vi "Get Serial Settings.vi"(8 "error in (no error)":errorcluster, 11 "Item Ref in":T4 format="%.0x") -> (0 "error out":errorcluster, 1 "baud rate":u32=9600, 2 "VISA resource name":refnum<visa-resource-name>, 3 "Item Ref out":T4 format="%.0x", 4 "parity (even)":T1=2 items=["None", "Odd", "Even", "Mark", "Space"], 5 "serial type":T2, 6 "Wire Mode":i32(ring)=-1 items=["Unknown"=-1, "RS485/Wire4"=0, "RS485/Wire2-EchoDTR"=1, "RS485/Wire2-CtrlDTR"=2, "RS485/Wire2-Auto"=3, "RS232/DTE"=128, "RS232/DCE"=129, "RS232/AUTO"=130], 7 "flow control (none)":T3 items=["None", "XON/XOFF", "RTS/CTS", "XON/XOFF & RTS/CTS", "DTR/DSR", "XON/XOFF & DTR/DSR"])   [LabVIEW 2020, in "Modbus Master System Explorer.lvlib"]
uses:
  Modbus Master System Explorer.lvlib
  <vilib>/NI VeriStand/Custom Device API/Custom Device Item Ref.ctl
  Shared/Controls/Flow Control.ctl
  Shared/Controls/Serial Type.ctl
  Shared/Controls/Parity.ctl
  Shared/Constants.vi
  <vilib>/NI VeriStand/Custom Device API/Get Item Property (String).vi
  <vilib>/NI VeriStand/Custom Device API/Get Item Property (U32).vi
  <vilib>/NI VeriStand/Custom Device API/Get Item Property (U16).vi
  <vilib>/NI VeriStand/Custom Device API/Get Item Property (I32).vi
  Shared/Modbus Master Shared.lvlib
  <vilib>/NI VeriStand/Custom Device API/Custom Device API.lvlib
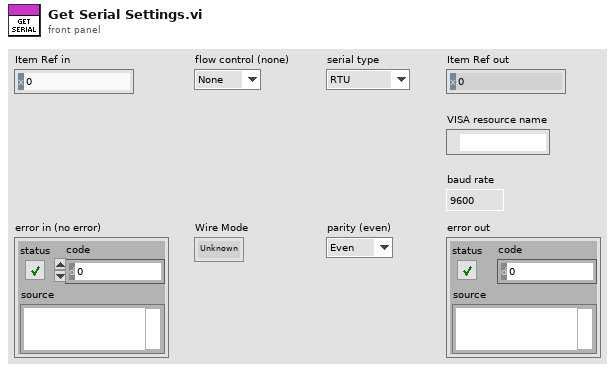
[diagram p1: front panel]
types:
  T1 = typedef "Modbus Master Shared.lvlib/Parity.ctl" = u16
  T2 = typedef "Modbus Master Shared.lvlib/Serial Type.ctl" = enum16{"RTU", "ASCII"}
  T3 = typedef "Modbus Master Shared.lvlib/Flow Control.ctl" = u16
  T4 = typedef "Custom Device API.lvlib/Custom Device Item Ref.ctl" = u64
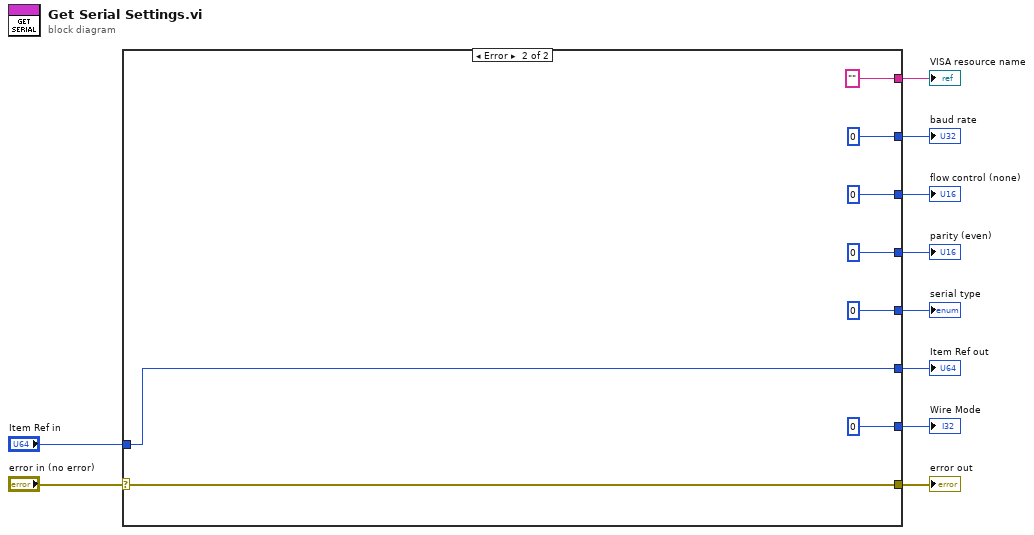
[diagram p0: block diagram]
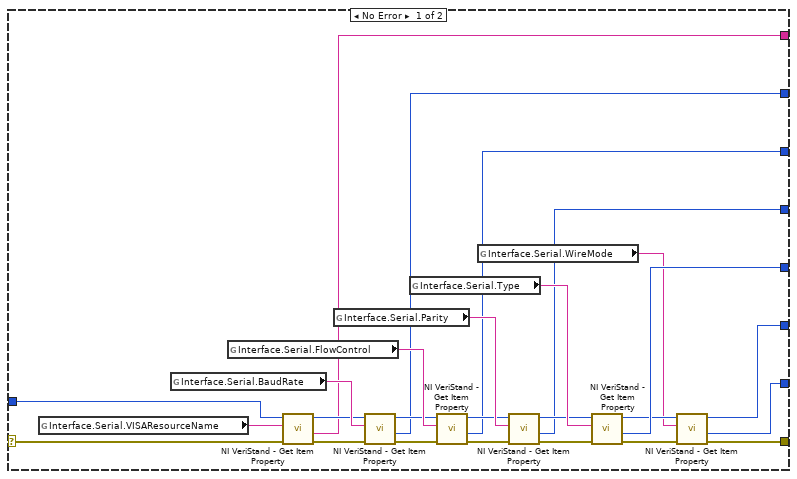
[diagram p2: hidden frame]
diagram:
  n1 = case shown="Error" "error in (no error)" {
    selector: "error in (no error)" -> [w24 w43]
    tunnel: [w11 w43] -> w10
    tunnel: [w14 w44] -> w9
    tunnel: "Item Ref in" -> [w23 w44]
    tunnel: [w21 "" ("Value")] -> w6
    tunnel: [w20 u32 0 ("Value")] -> w5
    tunnel: [w19 u16 0 ("Value")] -> w4
    tunnel: [w18 u16 0 ("Value")] -> w3
    tunnel: [w17 u16 0 ("Value")] -> w2
    tunnel: [w13 0 ("Value")] -> w1
    frame No Error {
      n2 = global read "Constants.vi" "Interface.Serial.VISAResourceName"() -> (w22:string)
      n3 = global read "Constants.vi" "Interface.Serial.BaudRate"() -> (w27:string)
      n4 = global read "Constants.vi" "Interface.Serial.FlowControl"() -> (w30:string)
      n5 = call-poly <vilib>:"NI VeriStand - Get Item Property.vi"("error in (no error)"=w24, "Property Name"=w22, "Item Ref in"=w23) -> ("error out"=w25:errorcluster, "Value"=w21:string, "Item Ref out"=w26:T4)  [unwired: 5 in, 1 out]
      n6 = global read "Constants.vi" "Interface.Serial.Parity"() -> (w33:string)
      n7 = call-poly <vilib>:"NI VeriStand - Get Item Property.vi"("error in (no error)"=w25, "Property Name"=w27, "Item Ref in"=w26) -> ("error out"=w28:errorcluster, "Value"=w20:u32, "Item Ref out"=w29:T4)  [unwired: 5 in, 1 out]
      n8 = global read "Constants.vi" "Interface.Serial.Type"() -> (w36:string)
      n9 = call-poly <vilib>:"NI VeriStand - Get Item Property.vi"("error in (no error)"=w28, "Property Name"=w30, "Item Ref in"=w29) -> ("error out"=w31:errorcluster, "Value"=w19:u16, "Item Ref out"=w32:T4)  [unwired: 5 in, 1 out]
      n10 = global read "Constants.vi" "Interface.Serial.WireMode"() -> (w12:string)
      n11 = call-poly <vilib>:"NI VeriStand - Get Item Property.vi"("error in (no error)"=w31, "Property Name"=w33, "Item Ref in"=w32) -> ("error out"=w34:errorcluster, "Value"=w18:u16, "Item Ref out"=w35:T4)  [unwired: 5 in, 1 out]
      n12 = call-poly <vilib>:"NI VeriStand - Get Item Property.vi"("error in (no error)"=w34, "Property Name"=w36, "Item Ref in"=w35) -> ("error out"=w15:errorcluster, "Value"=w17:u16, "Item Ref out"=w16:T4)  [unwired: 5 in, 1 out]
      n13 = call-poly <vilib>:"NI VeriStand - Get Item Property.vi"("error in (no error)"=w15, "Property Name"=w12, "Item Ref in"=w16) -> ("error out"=w11:errorcluster, "Value"=w13:i32, "Item Ref out"=w14:T4)  [unwired: 5 in, 1 out]
    }
    frame Error {
    }
  }
  "error out" <- w10
  "Item Ref out" <- w9
  "VISA resource name" <- w6
  "flow control (none)" <- w4
  "serial type" <- w2
  "parity (even)" <- w3
  "baud rate" <- w5
  "Wire Mode" <- w1
